vi "Stufentabelle ausgeben.vi"(9 "Neue Tabelle":T1) -> (1 "Tabelle":string[][](array[string]))   [LabVIEW 2020, in "Linearisierung v2.lvlib"]
uses:
  Linearisierung v2.lvlib
  Eingabetabelle.ctl
  Allgemein/allgemeine Sub-VIs.lvlib
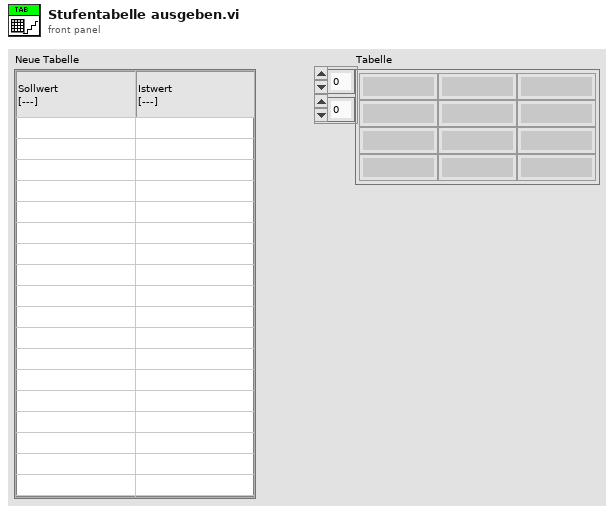
[diagram p1: front panel]
types:
  T1 = typedef "Linearisierung v2.lvlib/Eingabetabelle.ctl" = string[][]
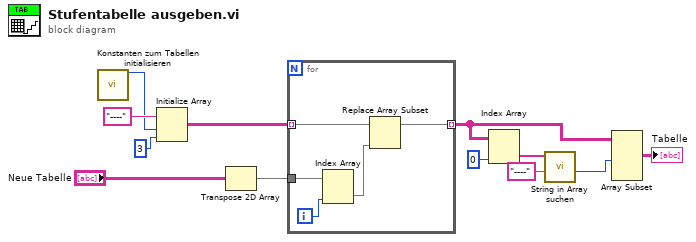
[diagram p0: block diagram]
diagram:
  n1 = call "Konstanten zum Tabellen initialisieren.vi"() -> ("Anzahl Gaskomponenten"=w1:i32)  [unwired: 13 in, 2 out]
  n2 = Initialize Array("----", w1, 3 ("Dimension")) -> (w6:string[][])
  n3 = Transpose 2D Array(2D array="Neue Tabelle") -> (transposed array=w2:T1)
  n4 = for {
    tunnel: w6 -> [w17] mode=indexing
    tunnel: w2 -> [w16]
    tunnel: [w13] -> w4 mode=indexing
    i -> [w15]
    n5 = Index Array(array=w16, index (col)=w15) -> (element=w14:string[])  [unwired: 1 in]
    n6 = Replace Array Subset(array=w17, new element=w14) -> (w13:string[])  [unwired: 1 in]
  }
  n7 = Index Array(array=w4, index (col)=0 ("Deaktivierter Index (Spalte)")) -> (element=w8:string[])  [unwired: 1 in]
  n8 = call "String in Array suchen.vi"("Nach String/Zeichen suchen (-)"="----", "String-Array"=w8) -> ("Index"=w10:i32)  [unwired: 7 in, 2 out]
  n9 = Array Subset(array=w4, length (row)=w10) -> (→"Tabelle":string[][])  [unwired: 3 in]
